vi "Convert StringArray To NumberArray.vi"(1 "String Array":string[](array[string])) -> (0 "Nuber Array":dbl[](array[numeric]))   [LabVIEW 2019]
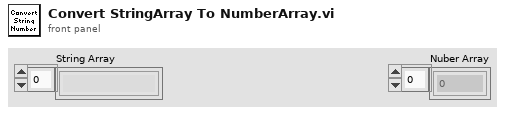
[diagram p1: front panel]
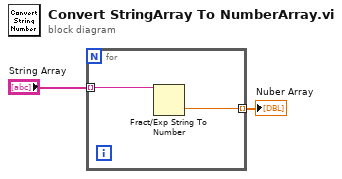
[diagram p0: block diagram]
diagram:
  n1 = for {
    tunnel: "String Array" -> [w4] mode=indexing
    tunnel: [w3] -> w1 mode=indexing
    n2 = Fract/Exp String To Number(string=w4) -> (number=w3:dbl)  [unwired: 3 in, 1 out]
  }
  "Nuber Array" <- w1
